vi "NIRFSG_SetOutput.vi"(8 "error in (no error)":errorcluster, 10 "output enabled":bool, 11 "RFSG Handle":refnum<k15>) -> (0 "error out":errorcluster)   [LabVIEW 2015]
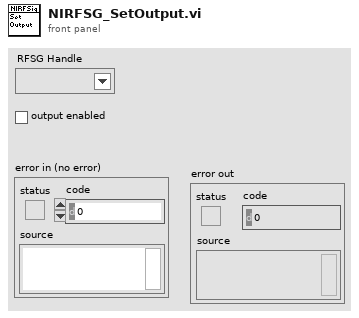
[diagram p1: front panel]
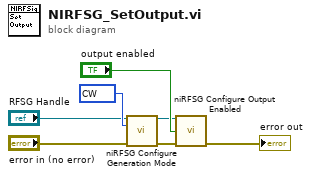
[diagram p0: block diagram]
diagram:
  w6 = 1000 items=["CW"=1000, "Arb Waveform"=1001, "Script"=1002] ("generation mode")
  n1 = call <instrlib>:"niRFSG Configure Generation Mode.vi"("instrument handle"="RFSG Handle", "generation mode"=w6, "error in"="error in (no error)") -> ("instrument handle out"=w5:refnum<k15>, "error out"=w4:errorcluster)  [unwired: 11 in]
  n2 = call <instrlib>:"niRFSG Configure Output Enabled.vi"("instrument handle"=w5, "output enabled"="output enabled", "error in"=w4) -> ("error out"=→"error out":errorcluster)  [unwired: 11 in, 1 out]
